vi "Day 6 - Wait For It.vi"() -> ()   [LabVIEW 2020, in "AoC 2023.lvlib"]
uses:
  AoC 2023.lvlib
panel:
  out "Puzzle Part-2 Answer":string
  out "Puzzle Answer":string
  in  "Puzzle Input":string="Time:      7  15   30\nDistance:  9  40  200"
  # "Enter the Puzzle Input and run the VI"
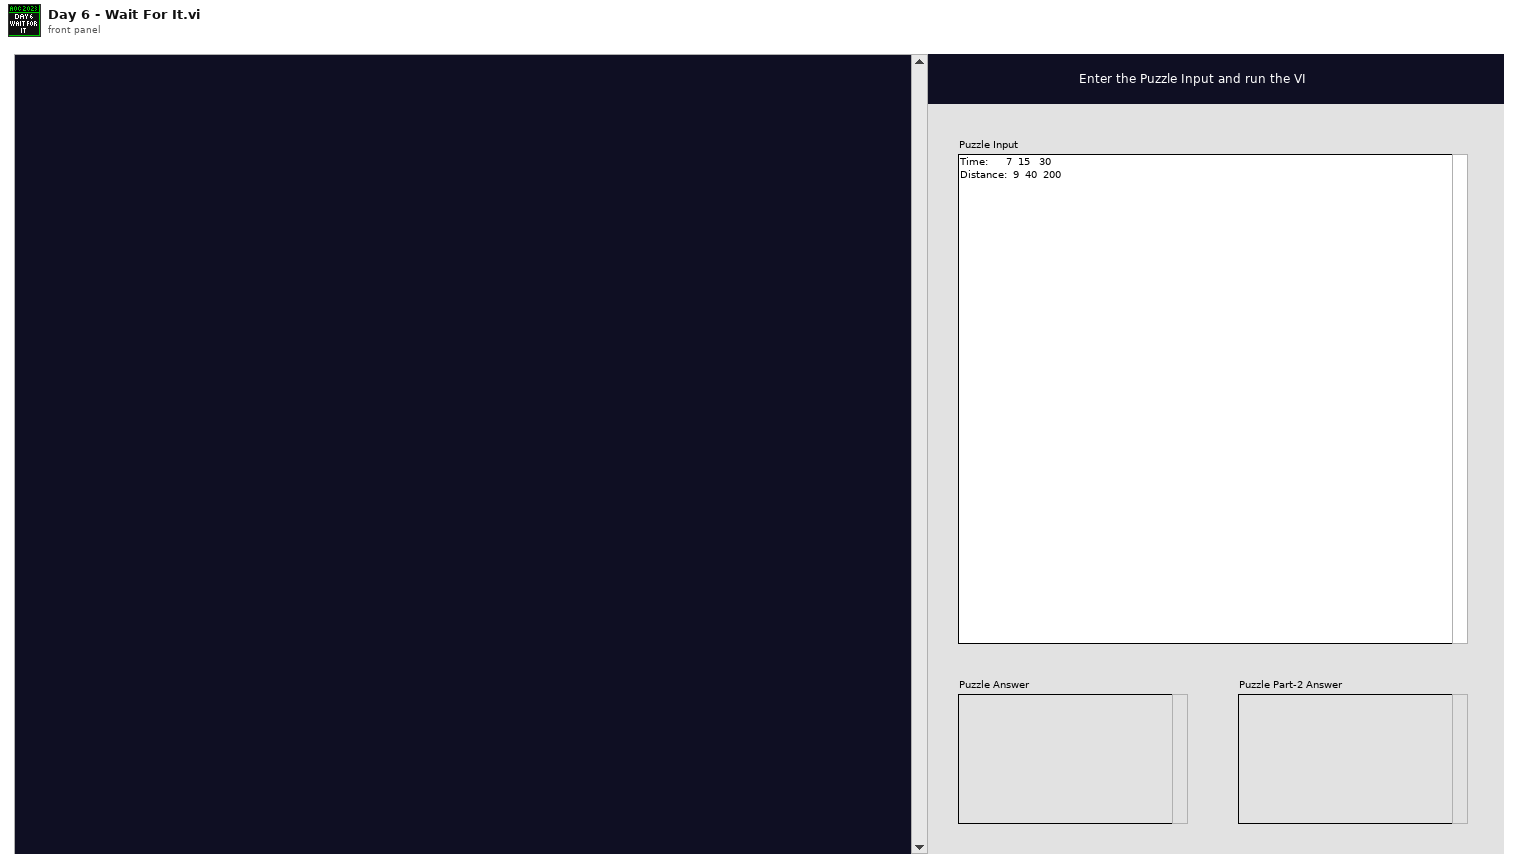
[diagram p1: front panel]
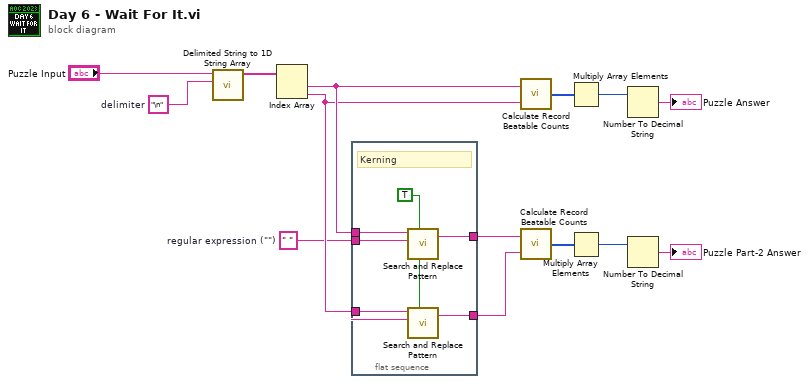
[diagram p0: block diagram]
diagram:
  w4 = " "  # regular expression ("")
  w11 = "\n"  # delimiter
  n1 = call <vilib>:"Delimited String to 1D String Array.vi"("delimiter"=w11, "delimited string"="Puzzle Input") -> ("string array"=w10:string[])  [unwired: 9 in]
  n2 = Index Array(array=w10) -> (element #1=w7:string, element #2=w5:string)  [unwired: 2 in]
  n3 = flat-sequence {
    tunnel: w7 -> [w20]
    tunnel: [w19] -> w6
    tunnel: w5 -> [w18]
    tunnel: w4 -> [w17]
    tunnel: [w15] -> w3
    frame #0 {
      w16 = TRUE
      # "Kerning"
      n4 = call <vilib>:"Search and Replace Pattern.vi"("string"=w20, "regular expression (\"\")"=w17, "replace all? (F)"=w16) -> ("result string"=w19:string)  [unwired: 2 in, 1 out]
      n5 = call <vilib>:"Search and Replace Pattern.vi"("string"=w18, "regular expression (\"\")"=w17, "replace all? (F)"=w16) -> ("result string"=w15:string)  [unwired: 2 in, 1 out]
    }
  }
  n6 = call "Calculate Record Beatable Counts.vi"("Distances"=w5, "Times"=w7) -> ("Record Beatable Counts"=w9:i32[])
  n7 = call "Calculate Record Beatable Counts.vi"("Distances"=w3, "Times"=w6) -> ("Record Beatable Counts"=w2:i32[])
  n8 = Multiply Array Elements(1:w9) -> (0:w8:i32)
  n9 = Multiply Array Elements(1:w2) -> (0:w1:i32)
  n10 = Number To Decimal String(number=w8) -> (decimal integer string=→"Puzzle Answer":string)  [unwired: 1 in]
  n11 = Number To Decimal String(number=w1) -> (decimal integer string=→"Puzzle Part-2 Answer":string)  [unwired: 1 in]
